vi "Moving Average.vi"() -> ()   [LabVIEW 2012]
uses:
  <vilib>/Analysis/baseanly.llb/Mean (DBL).vi
  <vilib>/Analysis/NI_AALBase.lvlib
panel:
  in  "SampleSize":u8=6
  out "Mean":dbl format="%0.2f"
  out "OutArray":dbl[](array[numeric])
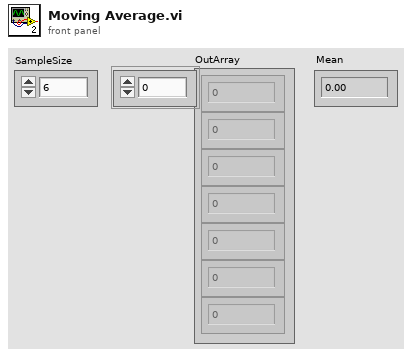
[diagram p1: front panel]
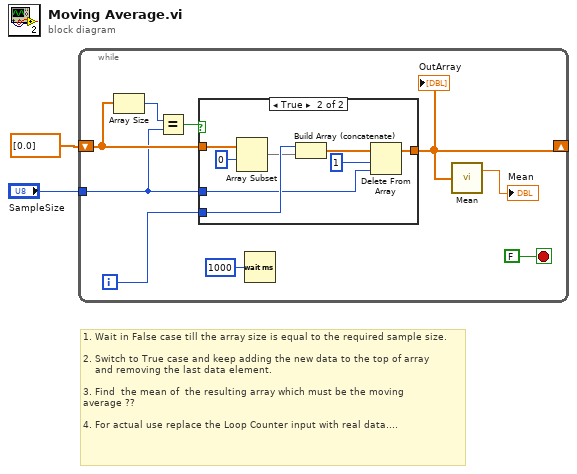
[diagram p0: block diagram]
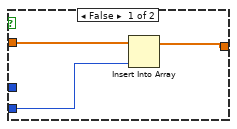
[diagram p2: hidden frame]
diagram:
  # "1. Wait in False case till the array size is equal to the required sample size.\n\n2. Switch to True case and keep adding the new data to the top of array \n    and removing the last data element. \n\n3. Find  the mean of  the resulting array which must be the moving \naverage ??\n\n4. For actual use replace the Loop Counter input with real data...."
  n1 = while {
    shift-right: [w5] -> _
    shift-left: dbl[] [0.0] -> [w9]
    tunnel: "SampleSize" -> [w3]
    i -> [w6]
    stop <- FALSE stop-if-true
    n2 = Array Size(array=w9) -> (size(s)=w8:i32)
    n3 = Equal?(x=w8, y=w3) -> (x = y?=w7:bool)
    n4 = case shown="True" w7 {
      tunnel: [w14 w17] -> w5
      tunnel: w9 -> [w13 w22]
      tunnel: w6 -> [w12 w20]
      tunnel: w3 -> [_ w15]
      frame False {
        n5 = Insert Into Array(array=w13, new element=w12) -> (w14:dbl[])  [unwired: 1 in]
      }
      frame True {
        n6 = Array Subset(array=w22, index=0) -> (w19:dbl[])  [unwired: 1 in]
        n7 = Build Array (concatenate)(w20, w19) -> (w18:dbl[])
        n8 = Delete From Array(array=w18, length=1, index=w15) -> (array with subset deleted=w17:dbl[])  [unwired: 1 out]
      }
    }
    "OutArray" <- w5
    n9 = Wait (ms)(milliseconds to wait=u32 1000) -> ()  [unwired: 1 out]
    n10 = call-poly <vilib>:"Mean.vi"("X"=w5) -> ("mean"=→"Mean":dbl)  [unwired: 1 out]
  }
